vi "Prepare Acyclic Tx Framing.vi"(8 "error in":errorcluster, 10 "channel number in":u8, 11 "board handle in":u8) -> (0 "error out":errorcluster, 2 "channel number out":u8, 3 "board handle out":u8)   [LabVIEW 2020, in "AIM ARINC 429 Hardware API.lvlib"]
uses:
  AIM ARINC 429 Hardware API.lvlib
  <instrlib>/AIM GmbH/_ARINC-429/AIM429LV.lvlib
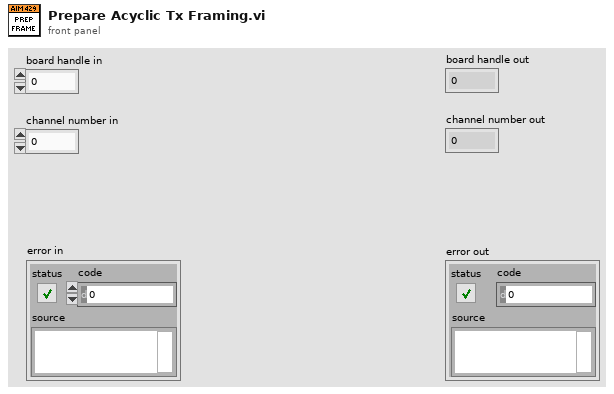
[diagram p1: front panel]
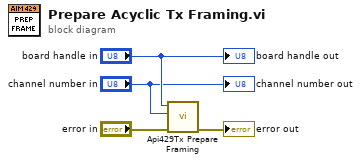
[diagram p0: block diagram]
diagram:
  n1 = call <instrlib>:"Api429Tx Prepare Framing.vi"("error in (no error)"="error in", "channel"="channel number in", "board_handle"="board handle in") -> ("error out"=→"error out":errorcluster)  [unwired: 8 in]
  "board handle out" <- "board handle in"
  "channel number out" <- "channel number in"
